vi "Close Device.vi"(8 "error in (no error)":errorcluster, 11 "Simulated in":refnum<class "Simulated-TS.lvclass">) -> (0 "error out":errorcluster, 3 "Simulated out":refnum<class "Simulated-TS.lvclass">)   [LabVIEW 2019, in "Simulated-TS.lvclass"]
uses:
  Simulated-TS.lvclass
  Abstract TranslationStage/Abstract TranslationStage.lvclass
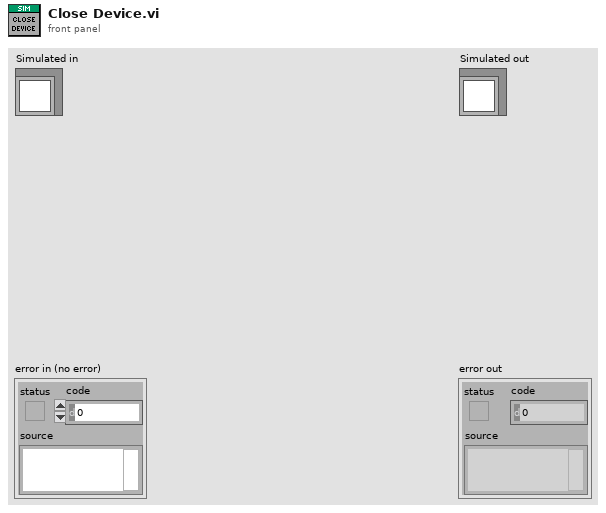
[diagram p1: front panel]
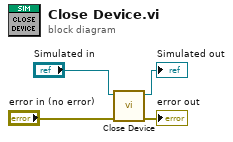
[diagram p0: block diagram]
diagram:
  n1 = call-parent "Close Device.vi"("error in (no error)"="error in (no error)", "Abstract TranslationStage in"="Simulated in") -> ("error out"=→"error out":errorcluster, "Abstract TranslationStage out"=→"Simulated out":refnum<class "Simulated-TS.lvclass">)  [unwired: 8 in]
